vi "SCLN_ResponseToClient.vi"(1 "error in (no error)":errorcluster, 2 "Message":string, 3 "Index for Response":i32) -> (0 "error out":errorcluster)   [LabVIEW 2015]
uses:
  SCLN_RW_Select.ctl
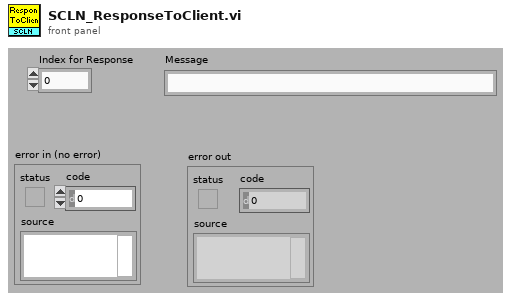
[diagram p1: front panel]
types:
  T1 = typedef "SCLN_RW_Select.ctl" = enum16{"Read", "Write"}
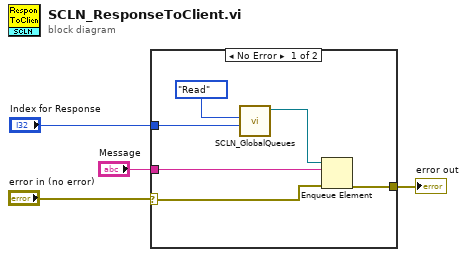
[diagram p0: block diagram]
diagram:
  n1 = case shown="No Error" "error in (no error)" {
    selector: "error in (no error)" -> [w5 w11]
    tunnel: [w7 w11] -> w3
    tunnel: "Index for Response" -> [w9 _]
    tunnel: "Message" -> [w6 _]
    frame No Error {
      n2 = call "SCLN_GlobalQueues.vi"("Element"=w9, "Operation"=SCLN_RW_Select."Read" ("GBL_RW")) -> ("Read QueueID"=w8:refnum<queue>)  [unwired: 6 in, 1 out]
      n3 = Enqueue Element(queue=w8, element=w6, error in (no error)=w5) -> (error out=w7:errorcluster)  [unwired: 1 in, 2 out]
    }
    frame Error {
    }
  }
  "error out" <- w3
